vi "editScriptCommandLimits.vi"() -> ()   [LabVIEW 2015]
doc: "Use this template to build a producer/consumer design pattern with events to produce queue items. Use this design pattern instead of the User Interface Event Handler pattern for user interfaces when you want to execute code asynchronously in response to an event without slowing the user interface responsiveness."
panel:
  out "Script Command":string
  in  "Back Up before saving":bool
  in  "Enter Line Number":u32
  in  "Save Line":bool
  in  "stop":bool
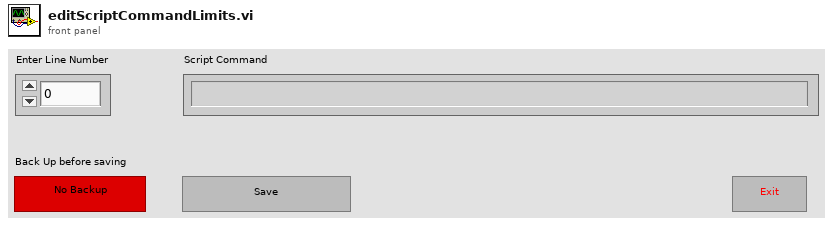
[diagram p1: front panel]
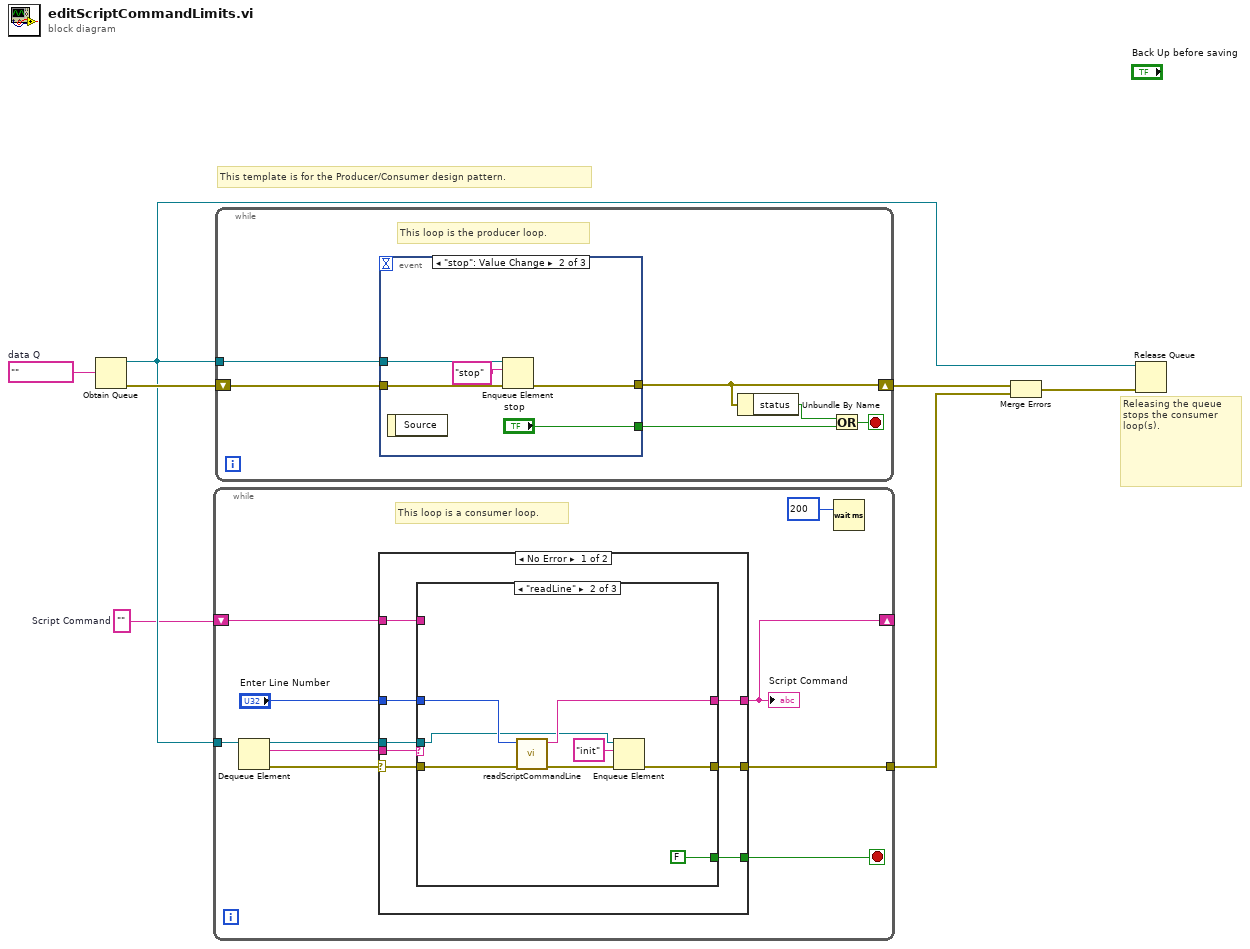
[diagram p0: block diagram]
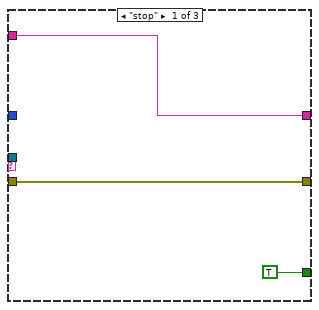
[diagram p2: hidden frame]
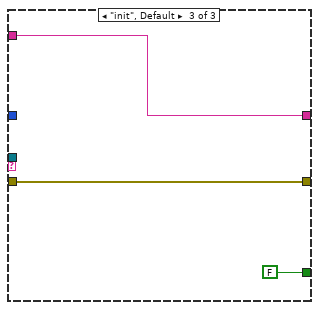
[diagram p3: hidden frame]
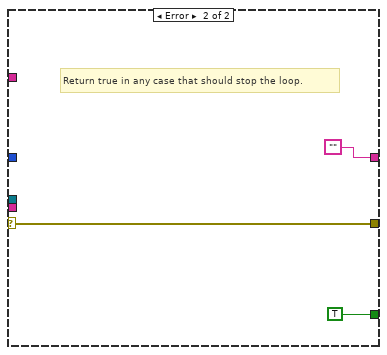
[diagram p4: hidden frame]
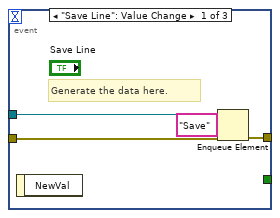
[diagram p5: hidden frame]
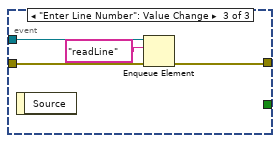
[diagram p6: hidden frame]
diagram:
  w1 = ""  # Script Command
  w5 = ""  # data Q
  # "Releasing the queue stops the consumer loop(s)."
  # "This template is for the Producer/Consumer design pattern."
  n1 = Obtain Queue(element data type=w5) -> (queue out=w4:refnum<queue>, error out=w7:errorcluster)  [unwired: 4 in, 1 out]
  n2 = while {
    tunnel: w4 -> [w17]
    tunnel: [w13] -> w2
    shift-right: [w10] -> _
    shift-left: w1 -> [w9]
    stop <- w14 stop-if-true
    # "This loop is a consumer loop."
    n3 = Dequeue Element(queue=w17) -> (queue out=w12:refnum<queue>, element=w15:string, error out=w16:errorcluster)  [unwired: 2 in, 1 out]
    n4 = case shown="No Error" w16 {
      selector: w16 -> [w23 w41]
      tunnel: w15 -> [w21 _]
      tunnel: [w25 TRUE] -> w14
      tunnel: [w22 w41] -> w13
      tunnel: w12 -> [w24 _]
      tunnel: [w20 ""] -> w10
      tunnel: w9 -> [w19 _]
      tunnel: "Enter Line Number" -> [w18 _]
      frame No Error {
        n5 = case shown="\"readLine\"" w21 {
          tunnel: [TRUE FALSE FALSE] -> w25
          tunnel: w24 -> [_ w29 _]
          tunnel: w23 -> [w27 w35 w38]
          tunnel: [w27 w31 w38] -> w22
          tunnel: [w26 w33 w37] -> w20
          tunnel: w19 -> [w26 _ w37]
          tunnel: w18 -> [_ w32 _]
          frame "stop" {
          }
          frame "readLine" {
            n6 = call "readScriptCommandLine.vi"("error in (no error)"=w35, "Enter Line Number"=w32) -> ("error out"=w34:errorcluster, "standard output"=w33:string)  [unwired: 8 in]
            n7 = Enqueue Element(queue=w29, element="init", error in (no error)=w34) -> (error out=w31:errorcluster)  [unwired: 1 in, 2 out]
          }
          frame "init", Default {
          }
        }
      }
      frame Error {
        # "Return true in any case that should stop the loop."
      }
    }
    "Script Command" <- w10
    n8 = Wait (ms)(milliseconds to wait=u32 200) -> ()  [unwired: 1 out]
  }
  n9 = while {
    shift-right: [w44] -> w6
    shift-left: w7 -> [w47]
    tunnel: w4 -> [w48]
    stop <- w45 stop-if-true
    # "This loop is the producer loop."
    n10 = event shown="[1] \"stop\": Value Change" {
      selector: _ -> [_ _ _]
      dyn-events: _ -> [_ _ _]
      timeout: _ -> [_ _ _]
      tunnel: w48 -> [w52 w53 w58]
      tunnel: w47 -> [w51 w55 w59]
      tunnel: [w50 w54 w60] -> w44
      tunnel: [_ "stop" _] -> w46
      event "Save Line": Value Change {
        # "Generate the data here."
        n11 = event-data() -> ()  [unwired: 1 in, 1 out]
        n12 = Enqueue Element(queue=w52, element="Save", error in (no error)=w51) -> (error out=w50:errorcluster)  [unwired: 1 in, 2 out]
      }
      event "stop": Value Change {
        n13 = event-data() -> ()  [unwired: 1 in, 1 out]
        n14 = Enqueue Element(queue=w53, element="stop", error in (no error)=w55) -> (error out=w54:errorcluster)  [unwired: 1 in, 2 out]
      }
      event "Enter Line Number": Value Change {
        n15 = event-data() -> ()  [unwired: 1 in, 1 out]
        n16 = Enqueue Element(queue=w58, element="readLine", error in (no error)=w59) -> (error out=w60:errorcluster)  [unwired: 1 in, 2 out]
      }
    }
    n17 = Unbundle By Name(w44) -> ("status"=w43:bool)
    n18 = Or(x=w43, y=w46) -> (x .or. y?=w45:bool)
  }
  n19 = Merge Errors(w6, w2) -> (w3:errorcluster)
  n20 = Release Queue(queue=w4, error in (no error)=w3) -> ()  [unwired: 1 in, 3 out]
